vi "hmi_shutdown.vi"(5 "hmi_references":T1, 8 "error in (no error)":errorcluster) -> (0 "error out":errorcluster)   [LabVIEW 2015, in "lv-post-installer-interface.lvlib"]
uses:
  lv-post-installer-interface.lvlib
  _controls/hmi_references.ctl
  _controls/tab_control.ctl
  _controls/navigation.ctl
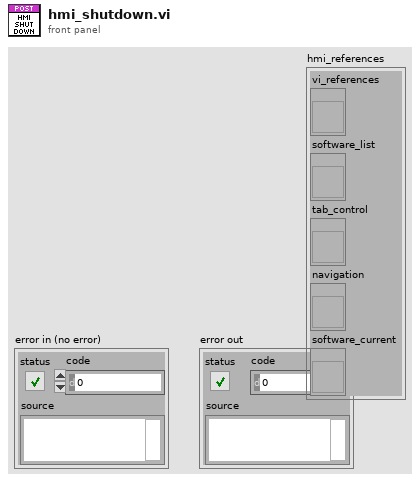
[diagram p1: front panel]
types:
  T1 = typedef "lv-post-installer-interface.lvlib/hmi_references.ctl" = cluster{"vi_references":refnum<vi>, "software_list":refnum<vi>, "tab_control":refnum<vi>, "navigation":refnum<vi>, "software_current":refnum<vi>}
  T2 = typedef "lv-post-installer-interface.lvlib/navigation.ctl" = enum32{"auxiliary", "automatic", "manual"}
  T3 = typedef "lv-post-installer-interface.lvlib/tab_control.ctl" = enum32{"automatic", "manual", "auxiliary"}
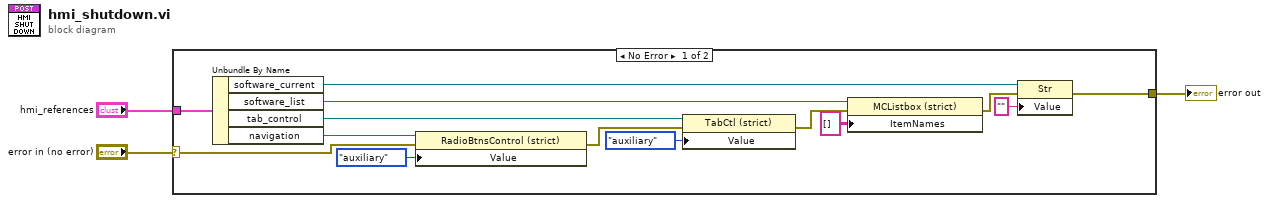
[diagram p0: block diagram]
diagram:
  n1 = case shown="No Error" "error in (no error)" {
    selector: "error in (no error)" -> [w14 w18]
    tunnel: [w4 w18] -> w2
    tunnel: "hmi_references" -> [w11 _]
    frame No Error {
      n2 = Unbundle By Name(w11) -> ("software_current"=w7:refnum<vi>, "software_list"=w10:refnum<vi>, "tab_control"=w9:refnum<vi>, "navigation"=w8:refnum<vi>)
      n3 = property on="Property Node" class="RadioBtnsControl (strict)"(reference=w8, error in=w14, "Value"=navigation."auxiliary" ("navigation")) -> (error out=w15:errorcluster)  [unwired: 1 out]
      n4 = property on="Property Node" class="TabCtl (strict)"(reference=w9, error in=w15, "Value"=tab_control."auxiliary" ("tab_control")) -> (error out=w13:errorcluster)  [unwired: 1 out]
      n5 = property on="Property Node" class="MCListbox (strict)"(reference=w10, error in=w13, "ItemNames"=string[][] [] ("Item Names")) -> (error out=w6:errorcluster)  [unwired: 1 out]
      n6 = property on="Property Node" class="Str"(reference=w7, error in=w6, "Value"="") -> (error out=w4:errorcluster)  [unwired: 1 out]
    }
    frame Error {
    }
  }
  "error out" <- w2
